vi "Compute Distance.vi"(8 "Y Image Resolution":i32, 9 "X Image Resolution":i32, 10 "Particle Scores":T1, 11 "Camera Type":enum16{"206", "1011"}(ring)) -> (1 "Center Target":bool, 2 "Target Center (-1 to 1)":cluster{"X":dbl, "Y":dbl}, 3 "Distance (ft)":dbl)   [LabVIEW 2013]
doc: "Using the camera lens information and the real world size of the target, use trig and simple math to determine the distance to the target. Also returns the location relative to the image center in a (-1 , 1) coordinate system that may be useful for steering the robot."
panel:
  in  "Camera view angle":dbl[](array[numeric])=[48.0, 43.5]
  # "Axis 206\nAxis M1011"
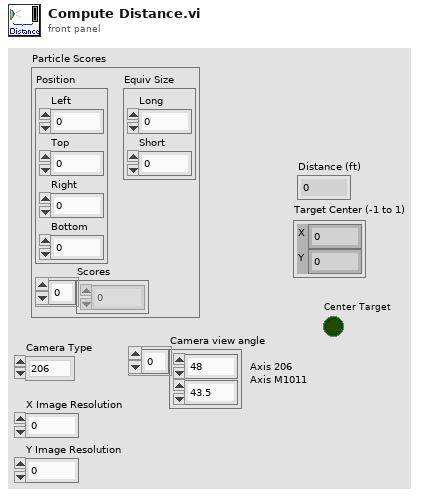
[diagram p1: front panel]
types:
  T1 = cluster{"Position":cluster{"Left":dbl, "Top":dbl, "Right":dbl, "Bottom":dbl}, "Scores":dbl[], "Equiv Size":cluster{"Long":dbl, "Short":dbl}}
  T2 = cluster{"X Image Resolution":i32, "Y Image Resolution":i32}
  T3 = cluster{"X Image Resolution":dbl, "Y Image Resolution":dbl}
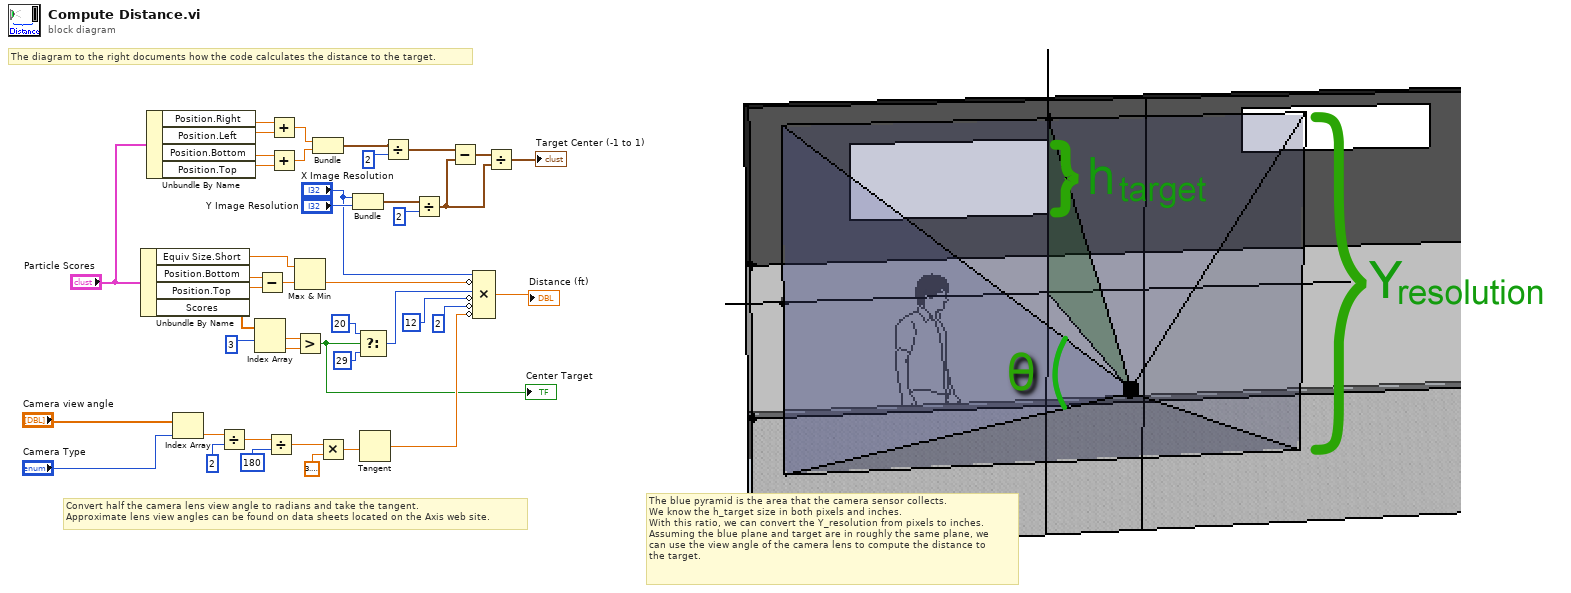
[diagram p0: block diagram]
diagram:
  # "The blue pyramid is the area that the camera sensor collects.\nWe know the h_target size in both pixels and inches.\nWith this ratio, we can convert the Y_resolution from pixels to inches.\nAssuming the blue plane and target are in roughly the same plane, we\ncan use the view angle of the camera lens to compute the distance to\nthe target."
  # "Convert half the camera lens view angle to radians and take the tangent.\nApproximate lens view angles can be found on data sheets located on the Axis web site."
  # "The diagram to the right documents how the code calculates the distance to the target."
  n1 = Unbundle By Name("Particle Scores") -> ("Equiv Size.Short"=w4:dbl, "Position.Bottom"=w34:dbl, "Position.Top"=w33:dbl, "Scores"=w17:dbl[])
  n2 = Unbundle By Name("Particle Scores") -> ("Position.Right"=w28:dbl, "Position.Left"=w29:dbl, "Position.Bottom"=w31:dbl, "Position.Top"=w30:dbl)
  n3 = Index Array(array="Camera view angle", index="Camera Type") -> (element=w40:dbl)
  n4 = Divide(x=w40, y=2) -> (x/y=w37:dbl)
  n5 = Index Array(array=w17, index #1=3) -> (element #1=w6:dbl, element #2=w15:dbl)  [unwired: 1 in]
  n6 = Subtract(x=w34, y=w33) -> (x-y=w3:dbl)
  n7 = Divide(x=w37, y=180) -> (x/y=w36:dbl)
  n8 = Add(x=w28, y=w29) -> (x+y=w26:dbl)
  n9 = Add(x=w31, y=w30) -> (x+y=w25:dbl)
  n10 = Max & Min(x=w4, y=w3) -> (min(x,y)=w2:dbl)  [unwired: 1 out]
  n11 = Greater?(x=w6, y=w15) -> (0:w7:bool)
  "Center Target" <- w7
  n12 = Bundle(w26, w25) -> (w22:cluster{dbl, dbl})  [unwired: 1 in]
  n13 = Multiply(x=w36, y=3.141592653589793) -> (x*y=w38:dbl)
  n14 = Bundle("X Image Resolution"="X Image Resolution", "Y Image Resolution"="Y Image Resolution") -> (w24:T2)  [unwired: 1 in]
  n15 = Select(t=20 ("Target Height (in)"), s=w7, f=29 ("Target Height (in)")) -> (s? t:f=w12:i32)
  n16 = Tangent(1:w38) -> (0:w10:dbl)
  n17 = Divide(x=w22, y=2) -> (x/y=w21:cluster{dbl, dbl})
  n18 = Divide(x=w24, y=2) -> (x/y=w19:T3)
  n19 = Subtract(x=w21, y=w19) -> (x-y=w20:cluster{dbl, dbl})
  n20 = Compound Arithmetic op=MULTIPLY("X Image Resolution", invert w2, w12, invert 12, invert 2, invert w10) -> (→"Distance (ft)":dbl)
  n21 = Divide(x=w20, y=w19) -> (x/y=→"Target Center (-1 to 1)":cluster{dbl, dbl})
